vi "Read Joystick State.vi"(8 "error in (no error)":errorcluster, 11 "Joystick in":refnum<class "Joystick.lvclass">) -> (0 "error out":errorcluster, 2 "Joystick State":T1, 3 "Joystick out":refnum<class "Joystick.lvclass">)   [LabVIEW 2014, in "Joystick.lvlib" / "Joystick.lvclass"]
uses:
  Joystick.lvclass
  Joystick State.ctl
  Button State.ctl
  Axis State.ctl
  Joystick.lvclass/Joystick.ctl
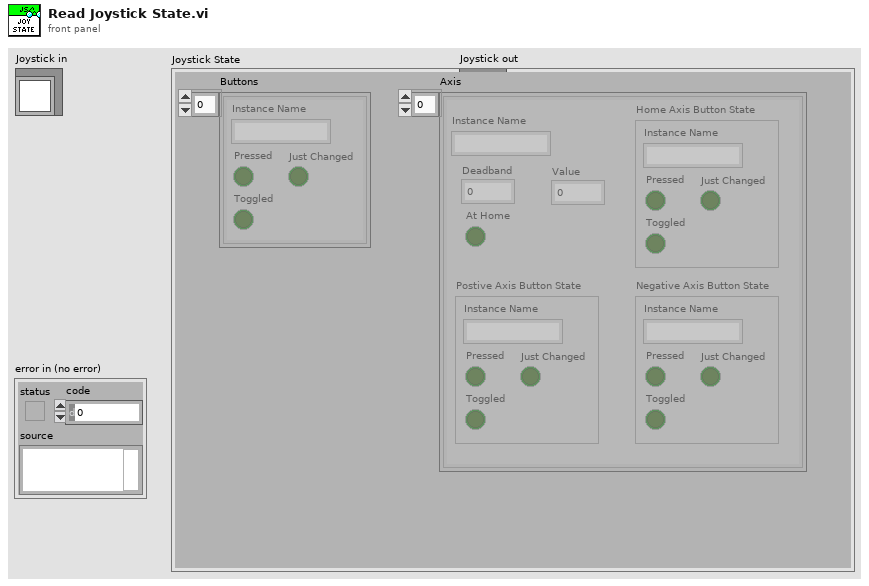
[diagram p1: front panel]
types:
  T1 = typedef "Joystick.lvlib/Joystick.lvclass/Joystick State.ctl" = cluster{"Buttons":T2[], "Axis":T3[]}
  T2 = typedef "Joystick.lvlib/Joystick.lvclass/Button State.ctl" = cluster{"Pressed":bool, "Instance Name":string, "Toggled":bool, "Just Changed":bool}
  T3 = typedef "Joystick.lvlib/Joystick.lvclass/Axis State.ctl" = cluster{"Instance Name":string, "Deadband":dbl, "Value":dbl, "At Home":bool, "Postive Axis Button State":T2, "Negative Axis Button State":T2, "Home Axis Button State":T2}
  T4 = enum16{"Critical", "Error", "Warning", "Informational", "Debug"}
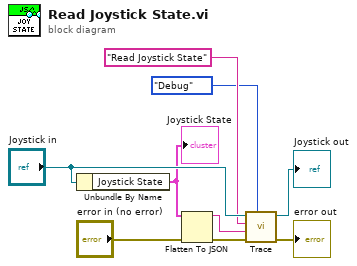
[diagram p0: block diagram]
diagram:
  n1 = Unbundle By Name("Joystick in") -> ("Joystick State"=w2:T1)
  "Joystick State" <- w2
  n2 = Flatten To JSON(anything=w2, error in (no error)="error in (no error)") -> (JSON string=w6:string, 11:w4:errorcluster)  [unwired: 1 in]
  n3 = call-dynamic "Trace.vi"("Trace Level"=T4."Debug", "error in (no error)"=w4, "System Message"=w6, "System Action"="Read Joystick State", "System Actor in"="Joystick in") -> ("error out"=→"error out":errorcluster, "System Actor out"=→"Joystick out":refnum<class "Joystick.lvclass">)  [unwired: 5 in]
